vi "GetCountdownAction.vi"(8 "PrevMode":T1(ring)=enum."Auto Disabled", 9 "PrevStatus":T2(ring), 10 "CurrentStatus":T2(ring), 11 "CurrentMode":T1(ring)=enum."Auto Disabled") -> (1 "Teleop?":bool, 2 "Action":T3)   [LabVIEW 2013]
doc: "Decides what action the timer should take. The possible actions are:\n-Start: when the robot switches from disabled to enabled\n-Reset: when the robot switches from enabled to disabled\n-Continue: when the robot remains in enabled mode\n-Idle: when the robot remains in disabled mode"
uses:
  CountdownAction.ctl
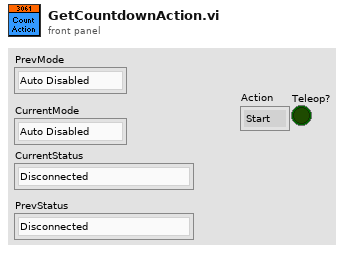
[diagram p1: front panel]
types:
  T1 = enum8{"Tele-Op Disabled", "Tele-Op Enabled", "Auto Disabled", "Auto Enabled", "Test Disabled", "Test Enabled", ""}
  T2 = enum8{"Disconnected", "E-Stop", "Disabled", "Enabled"}
  T3 = typedef "CountdownAction.ctl" = enum16{"Start", "Reset", "Continue", "Idle"}
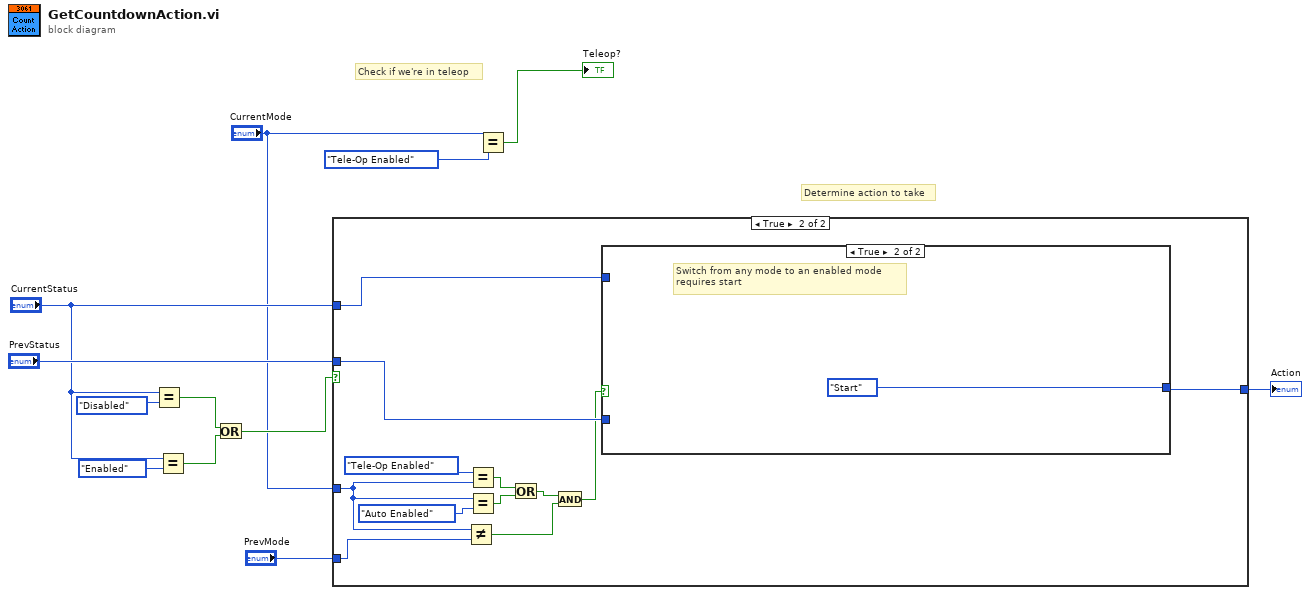
[diagram p0: block diagram]
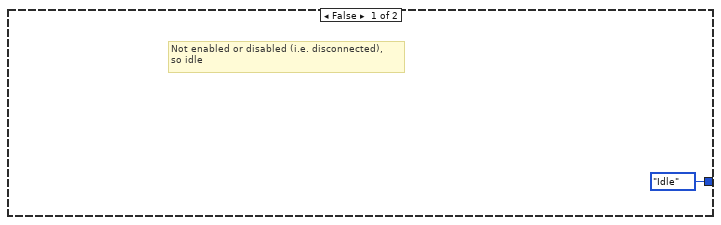
[diagram p2: hidden frame]
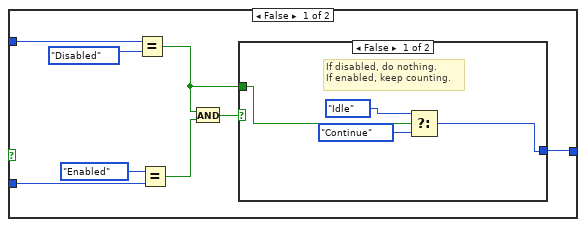
[diagram p3: hidden frame]
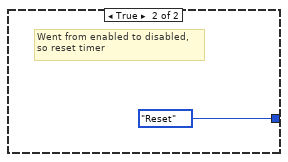
[diagram p4: hidden frame]
diagram:
  # "Determine action to take"
  # "Check if we're in teleop"
  n1 = Equal?(x="CurrentStatus", y=T2."Disabled") -> (x = y?=w5:bool)
  n2 = Equal?(x="CurrentStatus", y=T2."Enabled") -> (x = y?=w4:bool)
  n3 = Or(x=w5, y=w4) -> (x .or. y?=w3:bool)
  n4 = case shown="True" w3 {
    tunnel: [CountdownAction."Idle" ("Action") w25] -> w10
    tunnel: "CurrentStatus" -> [_ w24]
    tunnel: "PrevStatus" -> [_ w23]
    tunnel: "CurrentMode" -> [_ w17]
    tunnel: "PrevMode" -> [_ w16]
    frame False {
      # "Not enabled or disabled (i.e. disconnected), \nso idle"
    }
    frame True {
      n5 = Not Equal?(x=w17, y=w16) -> (x != y?=w15:bool)
      n6 = Equal?(x=T1."Tele-Op Enabled", y=w17) -> (x = y?=w21:bool)
      n7 = Equal?(x=w17, y=T1."Auto Enabled") -> (x = y?=w20:bool)
      n8 = Or(x=w21, y=w20) -> (x .or. y?=w19:bool)
      n9 = And(x=w19, y=w15) -> (x .and. y?=w14:bool)
      n10 = case shown="True" w14 {
        tunnel: [w28 CountdownAction."Start" ("Action")] -> w25
        tunnel: w24 -> [w27 _]
        tunnel: w23 -> [w33 _]
        frame False {
          n11 = Equal?(x=w27, y=T2."Disabled") -> (x = y?=w26:bool)
          n12 = Equal?(x=T2."Enabled", y=w33) -> (x = y?=w29:bool)
          n13 = And(x=w26, y=w29) -> (x .and. y?=w30:bool)
          n14 = case shown="False" w30 {
            tunnel: [w34 CountdownAction."Reset" ("Action")] -> w28
            tunnel: w26 -> [w37 _]
            frame False {
              # "If disabled, do nothing.\nIf enabled, keep counting."
              n15 = Select(t=CountdownAction."Idle" ("Action"), s=w37, f=CountdownAction."Continue") -> (s? t:f=w34:T3)
            }
            frame True {
              # "Went from enabled to disabled,\nso reset timer"
            }
          }
        }
        frame True {
          # "Switch from any mode to an enabled mode\nrequires start"
        }
      }
    }
  }
  "Action" <- w10
  n16 = Equal?(x="CurrentMode", y=T1."Tele-Op Enabled") -> (x = y?=→"Teleop?":bool)
